vi "Write Remote path.vi"(8 "error in (no error)":errorcluster, 10 "Remote path":string, 11 "[Test Case] Put and Get file in":refnum<class "[Test Case] Put and Get file.lvclass">) -> (0 "error out":errorcluster, 3 "[Test Case] Put and Get file out":refnum<class "[Test Case] Put and Get file.lvclass">)   [LabVIEW 2015, in "Tests.lvlib" / "[Test Case] Put and Get file.lvclass"]
uses:
  [Test Case] Put and Get file.lvclass
  [Test Case] Put and Get file.lvclass/[Test Case] Put and Get file.ctl
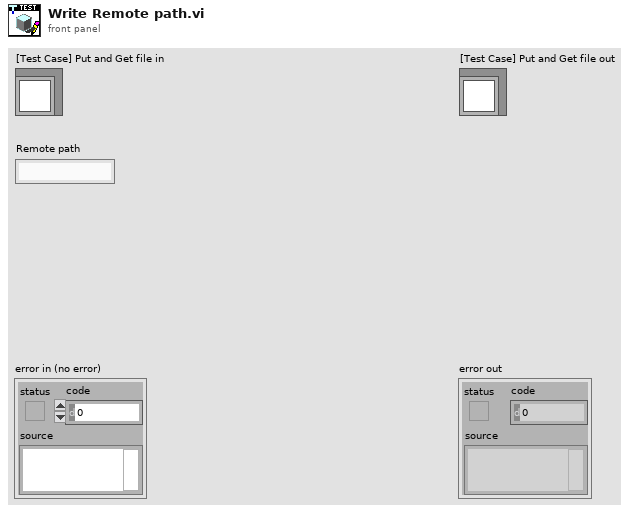
[diagram p1: front panel]
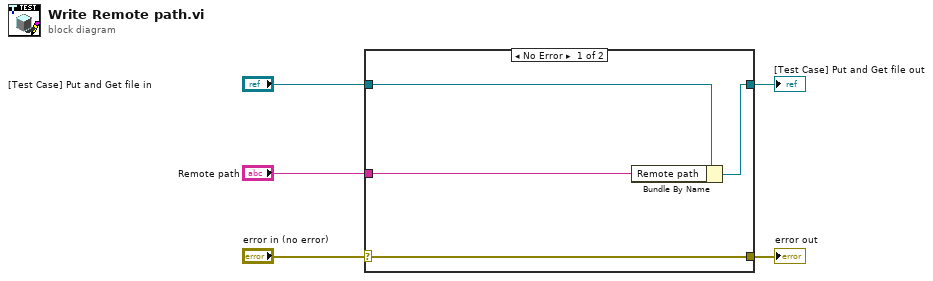
[diagram p0: block diagram]
diagram:
  n1 = case shown="No Error" "error in (no error)" {
    selector: "error in (no error)" -> [w9 w10]
    tunnel: [w9 w10] -> w4
    tunnel: [w7 w11] -> w2
    tunnel: "[Test Case] Put and Get file in" -> [w8 w11]
    tunnel: "Remote path" -> [w6 _]
    frame No Error {
      n2 = Bundle By Name(cluster=w8, "Remote path"=w6) -> (w7:refnum<class "[Test Case] Put and Get file.lvclass">)
    }
    frame Error {
    }
  }
  "error out" <- w4
  "[Test Case] Put and Get file out" <- w2
